vi "Create Pattern Script(Data).vi"(7 "Data Type":T1, 8 "error in (no error)":errorcluster, 10 "Data":u16, 11 "SPI Root Pattern Creator in":refnum<class "SPI Root Pattern Creator.lvclass">) -> (0 "error out":errorcluster, 2 "String":string, 3 "SPI Root Pattern Creator out":refnum<class "SPI Root Pattern Creator.lvclass">)   [LabVIEW 2018, in "SPI Root Pattern Creator.lvlib" / "SPI Root Pattern Creator.lvclass"]
uses:
  SPI Root Pattern Creator.lvclass
  Data Type.ctl
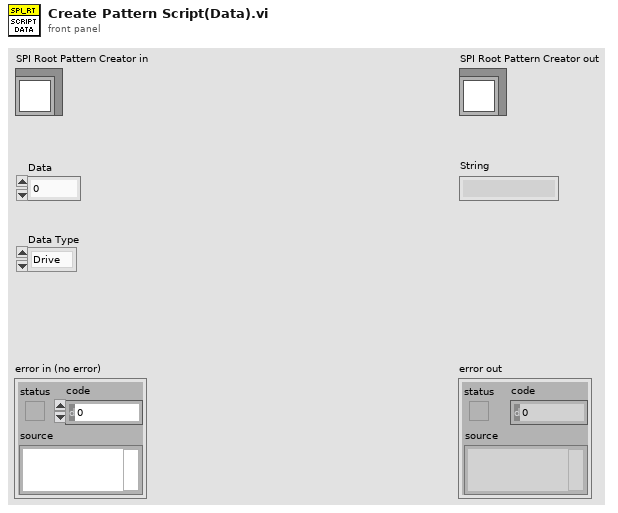
[diagram p1: front panel]
types:
  T1 = typedef "SPI Root Pattern Creator.lvlib/SPI Root Pattern Creator.lvclass/Data Type.ctl" = enum16{"Drive", "Compare", "Read"}
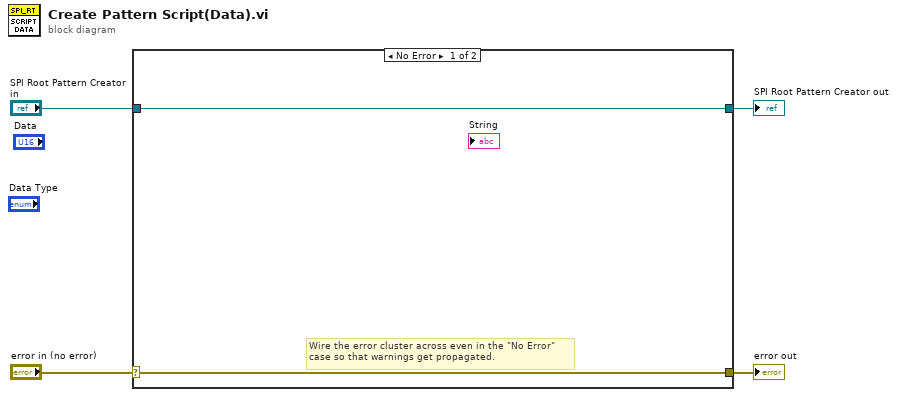
[diagram p0: block diagram]
diagram:
  n1 = case shown="No Error" "error in (no error)" {
    selector: "error in (no error)" -> [w5 w8]
    tunnel: [w5 w8] -> w3
    tunnel: [w6 w7] -> w1
    tunnel: "SPI Root Pattern Creator in" -> [w6 w7]
    frame No Error {
      # "Wire the error cluster across even in the \"No Error\"\ncase so that warnings get propagated."
    }
    frame Error {
    }
  }
  "error out" <- w3
  "SPI Root Pattern Creator out" <- w1
